vi "LEAPopen.vi"(8 "error in (no error)":errorcluster) -> (0 "error out":errorcluster, 3 ".NET Refnum out":refnum<k24>)   [LabVIEW 2017, in "LeapMotion.lvlib"]
uses:
  LeapMotion.lvlib
  C:/Users/snordinh/Desktop/LEAP-sign-language-test/LEAP-sign-language-test/LeapMotion/Dynamic Libraries/LeapCSharp.NET4.5.dll
  Dynamic Libraries/LeapCSharp.NET4.5.dll
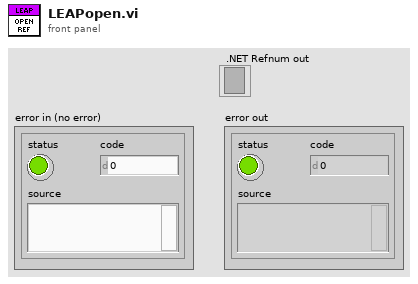
[diagram p1: front panel]
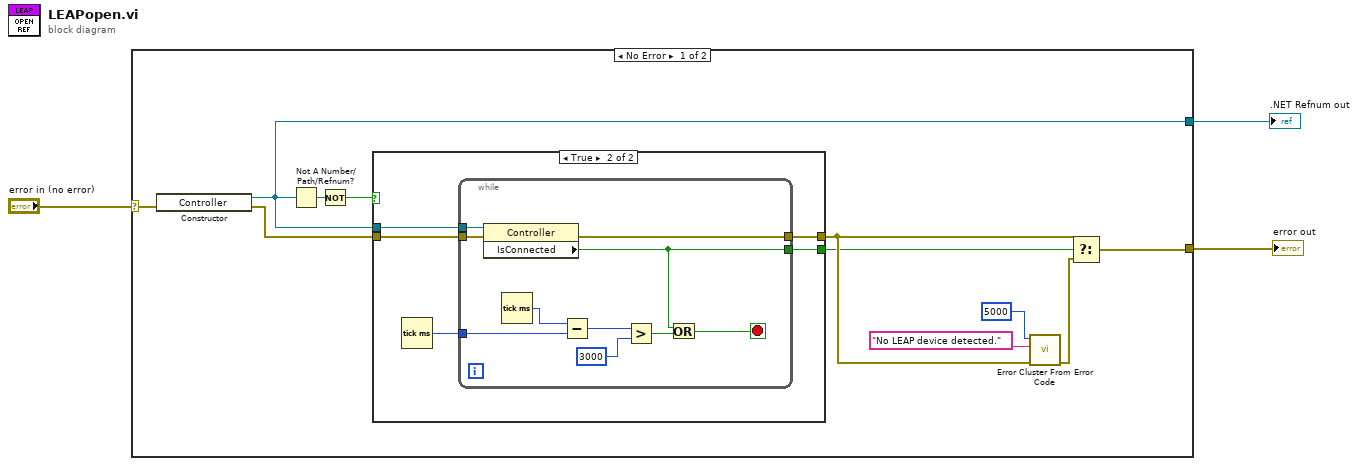
[diagram p0: block diagram]
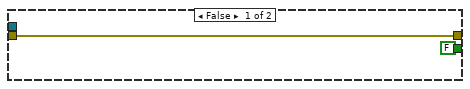
[diagram p2: hidden frame]
diagram:
  n1 = case shown="No Error" "error in (no error)" {
    selector: "error in (no error)" -> [w14 w32]
    tunnel: [w11 _] -> w2
    tunnel: [w4 w32] -> w3
    frame No Error {
      n2 = constructor class="Controller"(error in=w14) -> (reference out=w11:refnum<k24>, error out=w10:errorcluster)  [unwired: 2 in, 1 out]
      n3 = Not A Number/Path/Refnum?(number/path/refnum=w11) -> (NaN/Path/Refnum?=w13:bool)
      n4 = Not(x=w13) -> (.not. x?=w12:bool)
      n5 = case shown="True" w12 {
        tunnel: w11 -> [_ w21]
        tunnel: w10 -> [w15 w20]
        tunnel: [w15 w18] -> w6
        tunnel: [FALSE ("IsConnected") w17] -> w5
        frame False {
        }
        frame True {
          n6 = Tick Count (ms)() -> (millisecond timer value=w19:u32)
          n7 = while {
            tunnel: w21 -> [w31]
            tunnel: w20 -> [w30]
            tunnel: w19 -> [w27]
            tunnel: [w23] -> w18
            tunnel: [w22] -> w17
            stop <- w24 stop-if-true
            n8 = property class="Controller"(reference=w31, error in=w30) -> (error out=w23:errorcluster, "IsConnected"=w22:bool)  [unwired: 1 out]
            n9 = Tick Count (ms)() -> (millisecond timer value=w28:u32)
            n10 = Subtract(x=w28, y=w27) -> (x-y=w29:u32)
            n11 = Greater?(x=w29, y=u32 3000) -> (0:w25:bool)
            n12 = Or(x=w22, y=w25) -> (x .or. y?=w24:bool)
          }
        }
      }
      n13 = call <vilib>:"Error Cluster From Error Code.vi"("error in (no error)"=w6, "error message (\"\")"="No LEAP device detected." ("error message (\"\")"), "error code (0)"=5000) -> ("error out"=w7:errorcluster)  [unwired: 6 in]
      n14 = Select(t=w6, s=w5, f=w7) -> (s? t:f=w4:errorcluster)
    }
    frame Error {
    }
  }
  "error out" <- w3
  ".NET Refnum out" <- w2
